vi "pop_boolean.vi"(8 "error in (no error)":errorcluster, 11 "Lua in":refnum<class "Lua.lvclass">) -> (0 "error out":errorcluster, 2 "value":bool, 3 "Lua out":refnum<class "Lua.lvclass">)   [LabVIEW 2020, in "Lua for LabVIEW.lvlib" / "Lua.lvclass"]
doc: "Pop a boolean value from the stack."
uses:
  Lua.lvclass
  Lua.lvclass/Lua.ctl
  lib/lua.dll/types/lua_error_code_offset.vi
  lib/lua.dll/lua_settop.vi
  <vilib>/Utility/error.llb/Error Cluster From Error Code.vi
  lib/lua.dll/lua.dll.lvlib
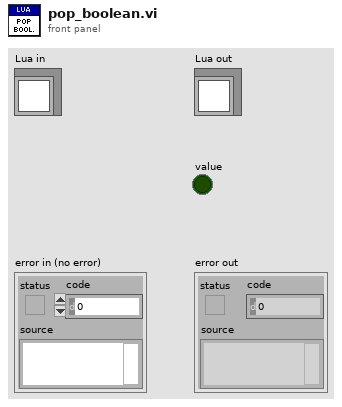
[diagram p1: front panel]
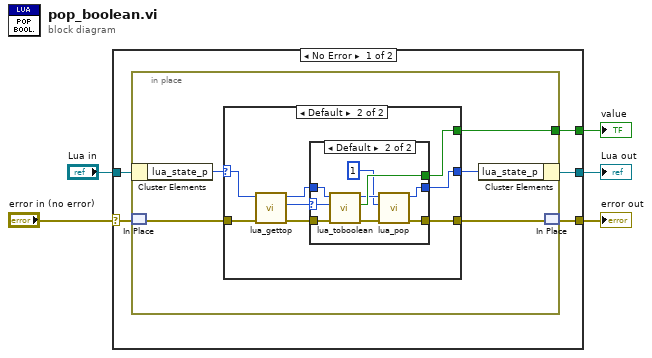
[diagram p0: block diagram]
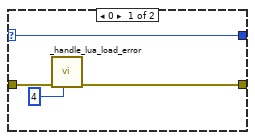
[diagram p2: hidden frame]
diagram:
  n1 = case shown="No Error" "error in (no error)" {
    selector: "error in (no error)" -> [w7 w40]
    tunnel: [w8 w40] -> w4
    tunnel: [w9 w39] -> w2
    tunnel: "Lua in" -> [w10 w39]
    tunnel: [w6 _] -> w1
    frame No Error {
      n2 = in-place {
        in-place-border: [w11] -> w6
        n3 = in-place-cluster #1(w10) -> ("lua_state_p"=w14:u64)
        n4 = in-place-match #2(w7) -> (w13:errorcluster)
        n5 = case shown="Default" w14 {
          selector: w14 -> [w19 w23]
          tunnel: [w19 w25] -> w15
          tunnel: w13 -> [w16 w24]
          tunnel: [w17 w26] -> w12
          tunnel: [_ w27] -> w11
          frame 0 {
            n6 = call "_handle_lua_load_error.vi"("lua_load errcode"=4, "error in (no error)"=w16) -> ("error out"=w17:errorcluster)  [unwired: 9 in]
          }
          frame Default {
            n7 = call "lua_gettop.vi"("error in (no error)"=w24, "lua_state_p"=w23) -> ("error out"=w21:errorcluster, "index"=w20:i32, "lua_state_p out"=w22:u64)  [unwired: 7 in]
            n8 = case shown="Default" w20 {
              selector: w20 -> [_ w30]
              tunnel: [_ w38] -> w27
              tunnel: [w28 w36] -> w26
              tunnel: [w29 w35] -> w25
              tunnel: w22 -> [w29 w32]
              tunnel: w21 -> [w28 w31]
              frame 0 {
              }
              frame Default {
                n9 = call "lua_toboolean.vi"("error in (no error)"=w31, "index"=w30, "lua_state_p"=w32) -> ("error out"=w37:errorcluster, "boolean"=w38:bool, "lua_state_p out"=w34:u64)  [unwired: 6 in]
                n10 = call "lua_pop.vi"("error in (no error)"=w37, "n"=1 ("index"), "lua_state_p"=w34) -> ("error out"=w36:errorcluster, "lua_state_p out"=w35:u64)  [unwired: 7 in]
              }
            }
          }
        }
        n11 = in-place-cluster #1("lua_state_p"=w15) -> (w9:refnum<class "Lua.lvclass">)
        n12 = in-place-match #2(w12) -> (w8:errorcluster)
      }
    }
    frame Error {
    }
  }
  "error out" <- w4
  "Lua out" <- w2
  "value" <- w1
